vi "__Test_MemoryToLvData.vi"() -> ()   [LabVIEW 2019]
uses:
  Memory Data Access.lvlib
panel:
  out "data_Cluster":T1
  out "data_Path":path
  out "data_Str":string
  out "data_DBL":dbl
  out "data_U32":u32
  out "data_I32":i32
  out "data_Waveform":waveform(dbl)
  out "data TimeStamp":timestamp
  out "data_Bool":bool
  out "data_ArrayWav":waveform(dbl)[](array[waveform])
  out "data_ArrayDBL":dbl[](array[numeric])
  out "data_ArrayStr":string[](array[string])
  in  "Enum":T2(ring)
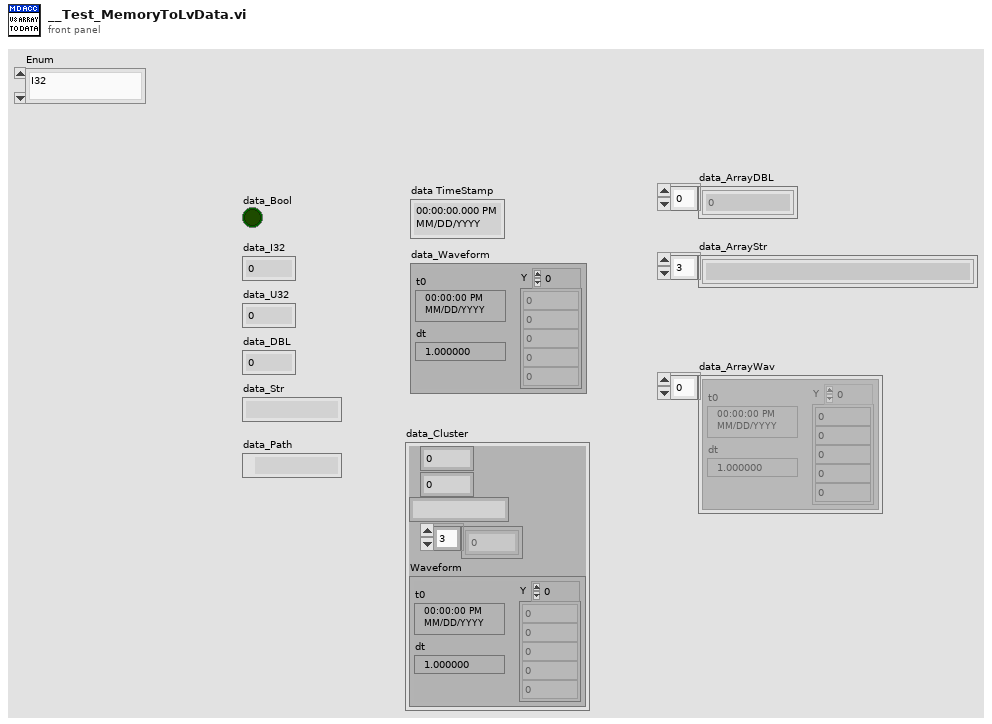
[diagram p1: front panel]
types:
  T1 = cluster{i32, dbl, string, dbl[], "Waveform":waveform(dbl)}
  T2 = enum16{"I32", "U32", "DBL", "String", "Cluster", "Array_Str", "Array_DBL", "Array_Waveform", "Bool", "TimeStamp", "Waveform", "Path"}
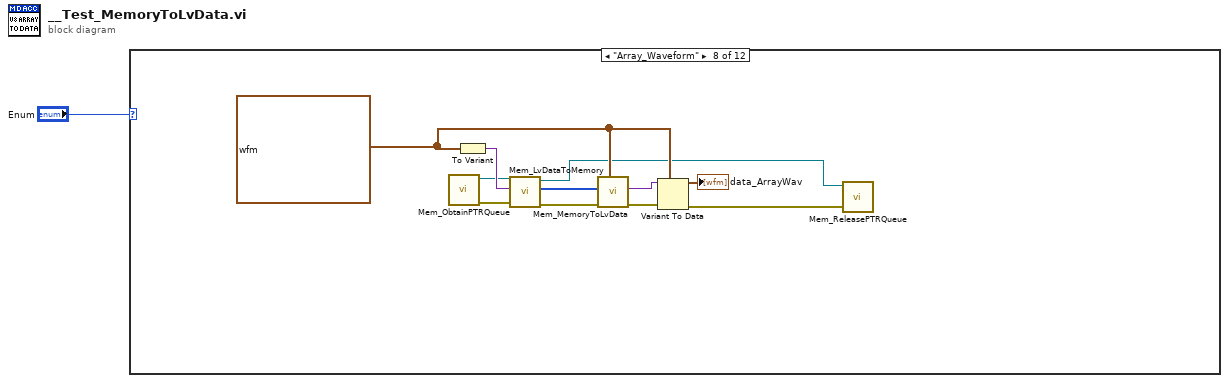
[diagram p0: block diagram]
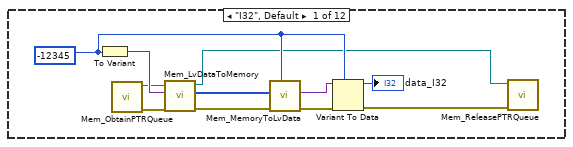
[diagram p2: hidden frame]
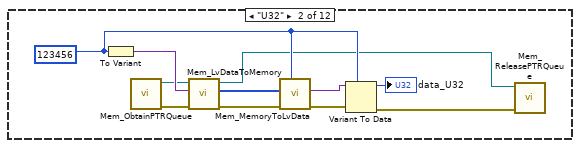
[diagram p3: hidden frame]
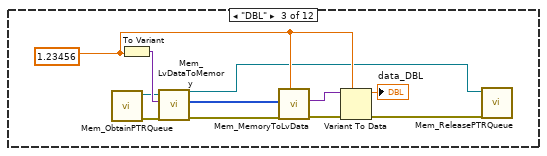
[diagram p4: hidden frame]
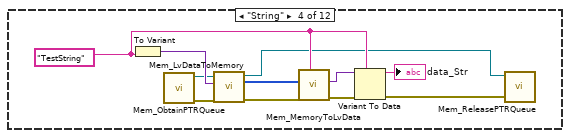
[diagram p5: hidden frame]
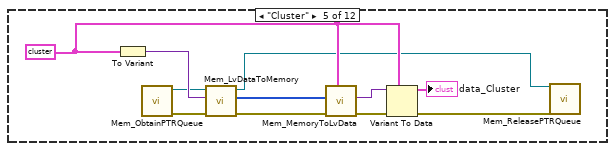
[diagram p6: hidden frame]
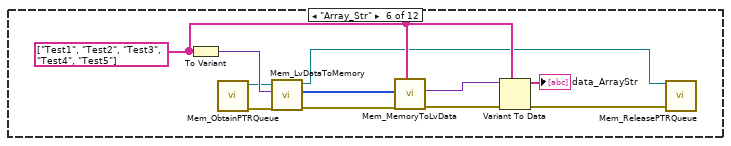
[diagram p7: hidden frame]
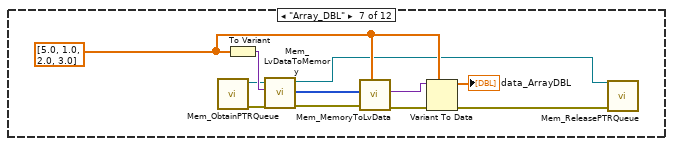
[diagram p8: hidden frame]
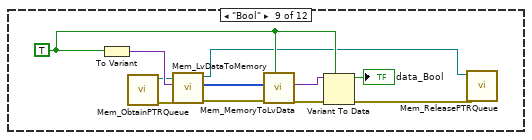
[diagram p9: hidden frame]
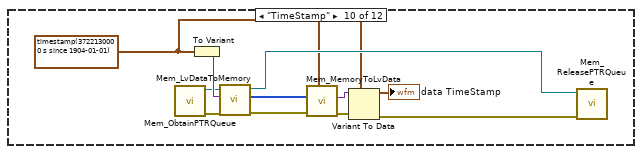
[diagram p10: hidden frame]
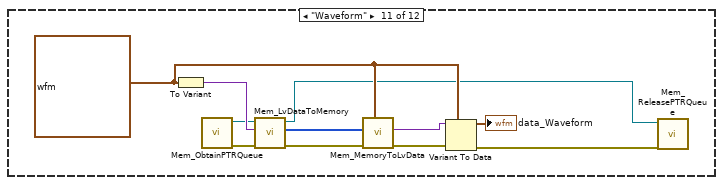
[diagram p11: hidden frame]
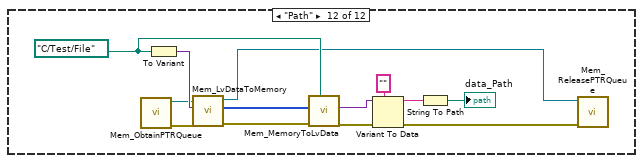
[diagram p12: hidden frame]
diagram:
  n1 = case shown="\"Array_Waveform\"" "Enum" {
    frame "I32", Default {
      w8 = -12345
      n2 = To Variant(anything=w8) -> (Variant=w12:variant)
      n3 = call "Mem_ObtainPTRQueue.vi"() -> ("error out"=w6:errorcluster, "queue out"=w5:refnum<queue>)  [unwired: 10 in]
      n4 = call "Mem_LvDataToMemory.vi"("error in (no error)"=w6, "Payload"=w12, "AddrQueueIn"=w5) -> ("error out"=w2:errorcluster, "ByteArray"=w11:u8[], "AddrQueueOut"=w4:refnum<queue>)  [unwired: 5 in, 1 out]
      n5 = call "Mem_MemoryToLvData.vi"("Type"=w8, "error in (no error)"=w2, "ByteArray"=w11) -> ("error out"=w10:errorcluster, "data"=w9:variant)  [unwired: 5 in, 2 out]
      n6 = Variant To Data(error in=w10, type=w8, Variant=w9) -> (data=→"data_I32":i32, error out=w3:errorcluster)
      n7 = call "Mem_ReleasePTRQueue.vi"("error in (no error)"=w3, "AddrQueueIn"=w4) -> ()  [unwired: 9 in, 1 out]
    }
    frame "U32" {
      w19 = u32 123456
      n8 = To Variant(anything=w19) -> (Variant=w23:variant)
      n9 = call "Mem_ObtainPTRQueue.vi"() -> ("error out"=w17:errorcluster, "queue out"=w16:refnum<queue>)  [unwired: 10 in]
      n10 = call "Mem_LvDataToMemory.vi"("error in (no error)"=w17, "Payload"=w23, "AddrQueueIn"=w16) -> ("error out"=w15:errorcluster, "ByteArray"=w22:u8[], "AddrQueueOut"=w14:refnum<queue>)  [unwired: 5 in, 1 out]
      n11 = call "Mem_MemoryToLvData.vi"("Type"=w19, "error in (no error)"=w15, "ByteArray"=w22) -> ("error out"=w20:errorcluster, "data"=w21:variant)  [unwired: 5 in, 2 out]
      n12 = Variant To Data(error in=w20, type=w19, Variant=w21) -> (data=→"data_U32":u32, error out=w13:errorcluster)
      n13 = call "Mem_ReleasePTRQueue.vi"("error in (no error)"=w13, "AddrQueueIn"=w14) -> ()  [unwired: 9 in, 1 out]
    }
    frame "DBL" {
      w30 = 1.23456
      n14 = call "Mem_ObtainPTRQueue.vi"() -> ("error out"=w28:errorcluster, "queue out"=w27:refnum<queue>)  [unwired: 10 in]
      n15 = To Variant(anything=w30) -> (Variant=w34:variant)
      n16 = call "Mem_LvDataToMemory.vi"("error in (no error)"=w28, "Payload"=w34, "AddrQueueIn"=w27) -> ("error out"=w26:errorcluster, "ByteArray"=w33:u8[], "AddrQueueOut"=w24:refnum<queue>)  [unwired: 5 in, 1 out]
      n17 = call "Mem_MemoryToLvData.vi"("Type"=w30, "error in (no error)"=w26, "ByteArray"=w33) -> ("error out"=w32:errorcluster, "data"=w31:variant)  [unwired: 5 in, 2 out]
      n18 = Variant To Data(error in=w32, type=w30, Variant=w31) -> (data=→"data_DBL":dbl, error out=w25:errorcluster)
      n19 = call "Mem_ReleasePTRQueue.vi"("error in (no error)"=w25, "AddrQueueIn"=w24) -> ()  [unwired: 9 in, 1 out]
    }
    frame "String" {
      w41 = "TestString"
      n20 = To Variant(anything=w41) -> (Variant=w45:variant)
      n21 = call "Mem_ObtainPTRQueue.vi"() -> ("error out"=w39:errorcluster, "queue out"=w38:refnum<queue>)  [unwired: 10 in]
      n22 = call "Mem_LvDataToMemory.vi"("error in (no error)"=w39, "Payload"=w45, "AddrQueueIn"=w38) -> ("error out"=w37:errorcluster, "ByteArray"=w44:u8[], "AddrQueueOut"=w36:refnum<queue>)  [unwired: 5 in, 1 out]
      n23 = call "Mem_MemoryToLvData.vi"("Type"=w41, "error in (no error)"=w37, "ByteArray"=w44) -> ("error out"=w43:errorcluster, "data"=w42:variant)  [unwired: 5 in, 2 out]
      n24 = Variant To Data(error in=w43, type=w41, Variant=w42) -> (data=→"data_Str":string, error out=w35:errorcluster)
      n25 = call "Mem_ReleasePTRQueue.vi"("error in (no error)"=w35, "AddrQueueIn"=w36) -> ()  [unwired: 9 in, 1 out]
    }
    frame "Cluster" {
      w52 = T1 {1245, 1.2345, "TestString", [0.0, 1.0, 2.0, 3.0], "Waveform"={"t0"=timestamp(3722126400 s since 1904-01-01), "dt"=1.0, "Y"=[1.0, 2.0, 3.0, 4.0]}}
      n26 = To Variant(anything=w52) -> (Variant=w56:variant)
      n27 = call "Mem_ObtainPTRQueue.vi"() -> ("error out"=w50:errorcluster, "queue out"=w49:refnum<queue>)  [unwired: 10 in]
      n28 = call "Mem_LvDataToMemory.vi"("error in (no error)"=w50, "Payload"=w56, "AddrQueueIn"=w49) -> ("error out"=w48:errorcluster, "ByteArray"=w55:u8[], "AddrQueueOut"=w47:refnum<queue>)  [unwired: 5 in, 1 out]
      n29 = call "Mem_MemoryToLvData.vi"("Type"=w52, "error in (no error)"=w48, "ByteArray"=w55) -> ("error out"=w53:errorcluster, "data"=w54:variant)  [unwired: 5 in, 2 out]
      n30 = Variant To Data(error in=w53, type=w52, Variant=w54) -> (data=→"data_Cluster":T1, error out=w46:errorcluster)
      n31 = call "Mem_ReleasePTRQueue.vi"("error in (no error)"=w46, "AddrQueueIn"=w47) -> ()  [unwired: 9 in, 1 out]
    }
    frame "Array_Str" {
      w64 = string[] ["Test1", "Test2", "Test3", "Test4", "Test5"]
      n32 = To Variant(anything=w64) -> (Variant=w67:variant)
      n33 = call "Mem_ObtainPTRQueue.vi"() -> ("error out"=w61:errorcluster, "queue out"=w60:refnum<queue>)  [unwired: 10 in]
      n34 = call "Mem_LvDataToMemory.vi"("error in (no error)"=w61, "Payload"=w67, "AddrQueueIn"=w60) -> ("error out"=w59:errorcluster, "ByteArray"=w66:u8[], "AddrQueueOut"=w58:refnum<queue>)  [unwired: 5 in, 1 out]
      n35 = call "Mem_MemoryToLvData.vi"("Type"=w64, "error in (no error)"=w59, "ByteArray"=w66) -> ("error out"=w62:errorcluster, "data"=w65:variant)  [unwired: 5 in, 2 out]
      n36 = Variant To Data(error in=w62, type=w64, Variant=w65) -> (data=→"data_ArrayStr":string[], error out=w57:errorcluster)
      n37 = call "Mem_ReleasePTRQueue.vi"("error in (no error)"=w57, "AddrQueueIn"=w58) -> ()  [unwired: 9 in, 1 out]
    }
    frame "Array_DBL" {
      w74 = dbl[] [5.0, 1.0, 2.0, 3.0]
      n38 = call "Mem_ObtainPTRQueue.vi"() -> ("error out"=w72:errorcluster, "queue out"=w71:refnum<queue>)  [unwired: 10 in]
      n39 = To Variant(anything=w74) -> (Variant=w78:variant)
      n40 = call "Mem_LvDataToMemory.vi"("error in (no error)"=w72, "Payload"=w78, "AddrQueueIn"=w71) -> ("error out"=w69:errorcluster, "ByteArray"=w77:u8[], "AddrQueueOut"=w70:refnum<queue>)  [unwired: 5 in, 1 out]
      n41 = call "Mem_MemoryToLvData.vi"("Type"=w74, "error in (no error)"=w69, "ByteArray"=w77) -> ("error out"=w75:errorcluster, "data"=w76:variant)  [unwired: 5 in, 2 out]
      n42 = Variant To Data(error in=w75, type=w74, Variant=w76) -> (data=→"data_ArrayDBL":dbl[], error out=w68:errorcluster)
      n43 = call "Mem_ReleasePTRQueue.vi"("error in (no error)"=w68, "AddrQueueIn"=w70) -> ()  [unwired: 9 in, 1 out]
    }
    frame "Array_Waveform" {
      w85 = waveform(dbl)[] [{"t0"=timestamp(3705278400 s since 1904-01-01), "dt"=1.0, "Y"=[1.0, 2.0, 3.0]}, {"t0"=timestamp(3705278400 s since 1904-01-01), "dt"=1.0, "Y"=[4.0, 5.0, 6.0]}]
      n44 = call "Mem_ObtainPTRQueue.vi"() -> ("error out"=w83:errorcluster, "queue out"=w82:refnum<queue>)  [unwired: 10 in]
      n45 = To Variant(anything=w85) -> (Variant=w89:variant)
      n46 = call "Mem_LvDataToMemory.vi"("error in (no error)"=w83, "Payload"=w89, "AddrQueueIn"=w82) -> ("error out"=w81:errorcluster, "ByteArray"=w88:u8[], "AddrQueueOut"=w80:refnum<queue>)  [unwired: 5 in, 1 out]
      n47 = call "Mem_MemoryToLvData.vi"("Type"=w85, "error in (no error)"=w81, "ByteArray"=w88) -> ("error out"=w87:errorcluster, "data"=w86:variant)  [unwired: 5 in, 2 out]
      n48 = Variant To Data(error in=w87, type=w85, Variant=w86) -> (data=→"data_ArrayWav":waveform(dbl)[], error out=w79:errorcluster)
      n49 = call "Mem_ReleasePTRQueue.vi"("error in (no error)"=w79, "AddrQueueIn"=w80) -> ()  [unwired: 9 in, 1 out]
    }
    frame "Bool" {
      w96 = TRUE
      n50 = To Variant(anything=w96) -> (Variant=w100:variant)
      n51 = call "Mem_ObtainPTRQueue.vi"() -> ("error out"=w94:errorcluster, "queue out"=w93:refnum<queue>)  [unwired: 10 in]
      n52 = call "Mem_LvDataToMemory.vi"("error in (no error)"=w94, "Payload"=w100, "AddrQueueIn"=w93) -> ("error out"=w92:errorcluster, "ByteArray"=w99:u8[], "AddrQueueOut"=w91:refnum<queue>)  [unwired: 5 in, 1 out]
      n53 = call "Mem_MemoryToLvData.vi"("Type"=w96, "error in (no error)"=w92, "ByteArray"=w99) -> ("error out"=w97:errorcluster, "data"=w98:variant)  [unwired: 5 in, 2 out]
      n54 = Variant To Data(error in=w97, type=w96, Variant=w98) -> (data=→"data_Bool":bool, error out=w90:errorcluster)
      n55 = call "Mem_ReleasePTRQueue.vi"("error in (no error)"=w90, "AddrQueueIn"=w91) -> ()  [unwired: 9 in, 1 out]
    }
    frame "TimeStamp" {
      w101 = timestamp(3722130000 s since 1904-01-01)
      n56 = call "Mem_ObtainPTRQueue.vi"() -> ("error out"=w106:errorcluster, "queue out"=w105:refnum<queue>)  [unwired: 10 in]
      n57 = To Variant(anything=w101) -> (Variant=w111:variant)
      n58 = call "Mem_LvDataToMemory.vi"("error in (no error)"=w106, "Payload"=w111, "AddrQueueIn"=w105) -> ("error out"=w104:errorcluster, "ByteArray"=w110:u8[], "AddrQueueOut"=w103:refnum<queue>)  [unwired: 5 in, 1 out]
      n59 = call "Mem_MemoryToLvData.vi"("Type"=w101, "error in (no error)"=w104, "ByteArray"=w110) -> ("error out"=w109:errorcluster, "data"=w108:variant)  [unwired: 5 in, 2 out]
      n60 = Variant To Data(error in=w109, type=w101, Variant=w108) -> (data=→"data TimeStamp":timestamp, error out=w102:errorcluster)
      n61 = call "Mem_ReleasePTRQueue.vi"("error in (no error)"=w102, "AddrQueueIn"=w103) -> ()  [unwired: 9 in, 1 out]
    }
    frame "Waveform" {
      w118 = waveform(dbl) {"t0"=timestamp(3722126400 s since 1904-01-01), "dt"=1.0, "Y"=[1.0, 2.0, 3.0, 4.0]} ("Waveform")
      n62 = To Variant(anything=w118) -> (Variant=w122:variant)
      n63 = call "Mem_ObtainPTRQueue.vi"() -> ("error out"=w116:errorcluster, "queue out"=w115:refnum<queue>)  [unwired: 10 in]
      n64 = call "Mem_LvDataToMemory.vi"("error in (no error)"=w116, "Payload"=w122, "AddrQueueIn"=w115) -> ("error out"=w114:errorcluster, "ByteArray"=w121:u8[], "AddrQueueOut"=w113:refnum<queue>)  [unwired: 5 in, 1 out]
      n65 = call "Mem_MemoryToLvData.vi"("Type"=w118, "error in (no error)"=w114, "ByteArray"=w121) -> ("error out"=w119:errorcluster, "data"=w120:variant)  [unwired: 5 in, 2 out]
      n66 = Variant To Data(error in=w119, type=w118, Variant=w120) -> (data=→"data_Waveform":waveform(dbl), error out=w112:errorcluster)
      n67 = call "Mem_ReleasePTRQueue.vi"("error in (no error)"=w112, "AddrQueueIn"=w113) -> ()  [unwired: 9 in, 1 out]
    }
    frame "Path" {
      w131 = path "C:/Test/File"
      n68 = call "Mem_ObtainPTRQueue.vi"() -> ("error out"=w127:errorcluster, "queue out"=w126:refnum<queue>)  [unwired: 10 in]
      n69 = To Variant(anything=w131) -> (Variant=w135:variant)
      n70 = call "Mem_LvDataToMemory.vi"("error in (no error)"=w127, "Payload"=w135, "AddrQueueIn"=w126) -> ("error out"=w125:errorcluster, "ByteArray"=w134:u8[], "AddrQueueOut"=w124:refnum<queue>)  [unwired: 5 in, 1 out]
      n71 = call "Mem_MemoryToLvData.vi"("Type"=w131, "error in (no error)"=w125, "ByteArray"=w134) -> ("error out"=w133:errorcluster, "data"=w132:variant)  [unwired: 5 in, 2 out]
      n72 = Variant To Data(error in=w133, type="", Variant=w132) -> (data=w129:string, error out=w123:errorcluster)
      n73 = String To Path(string=w129) -> (path=→"data_Path":path)
      n74 = call "Mem_ReleasePTRQueue.vi"("error in (no error)"=w123, "AddrQueueIn"=w124) -> ()  [unwired: 9 in, 1 out]
    }
  }
